vi "New Nested Logger Normal.vi"(8 "error in (no error)":errorcluster, 11 "caller actor in":refnum<class "Actor.lvclass">) -> (0 "error out":errorcluster, 2 "logger normal":refnum<class "Logger Normal.lvclass">, 3 "caller actor out":refnum<class "Actor.lvclass">)   [LabVIEW 2020, in "Logger Normal.lvlib" / "Logger Normal.lvclass"]
uses:
  Logger Normal.lvclass
  <vilib>/ActorFramework/Actor/Actor.lvclass
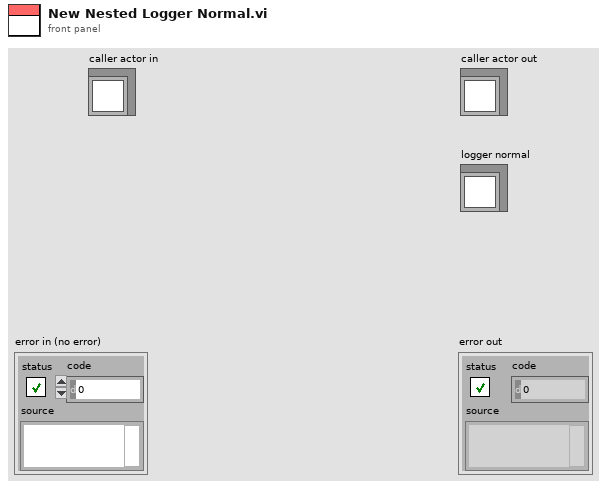
[diagram p1: front panel]
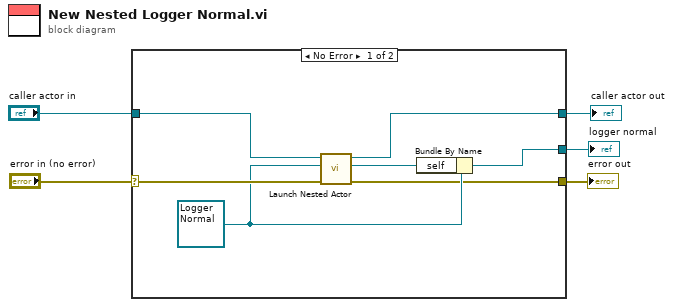
[diagram p0: block diagram]
diagram:
  n1 = case shown="No Error" "error in (no error)" {
    selector: "error in (no error)" -> [w12 w14]
    tunnel: [w9 w14] -> w4
    tunnel: [w8 _] -> w3
    tunnel: "caller actor in" -> [w7 w13]
    tunnel: [w6 w13] -> w1
    frame No Error {
      w11 = refnum<class "Logger Normal.lvclass"> refnum ("Logger Normal in")
      n2 = call <vilib>:"Launch Nested Actor.vi"("error in (no error)"=w12, "Nested Actor"=w11, "Caller Actor in"=w7) -> ("error out"=w9:errorcluster, "Nested Actor's Enqueuer"=w10:refnum<class "Message Enqueuer.lvclass">, "Caller Actor out"=w6:refnum<class "Actor.lvclass">)  [unwired: 6 in]
      n3 = Bundle By Name(cluster=w11, "self"=w10) -> (w8:refnum<class "Logger Normal.lvclass">)
    }
    frame Error {
    }
  }
  "error out" <- w4
  "logger normal" <- w3
  "caller actor out" <- w1
